vi "VG_DeltaTcell.vi"() -> ()   [LabVIEW 2020]
panel:
  out "DeltaTcell":dbl
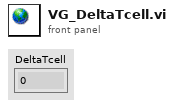
[diagram p1: front panel]
diagram:
